vi "CPP_BandLimitBoost.vi"(0 "CutoffFrequencyUsed":dbl=15.0, 3 "CutoffIndex":dbl, 4 "AmplitudeBoost":dbl[](array[numeric])) -> (1 "BandLimitedBoost":dbl[](array[numeric]))   [LabVIEW 2011]
uses:
  <vilib>/Analysis/NI_AALBase.lvlib
panel:
  in  "dF":dbl=0.06103515625
  in  "Combo Box":string(combo)="Cosine"
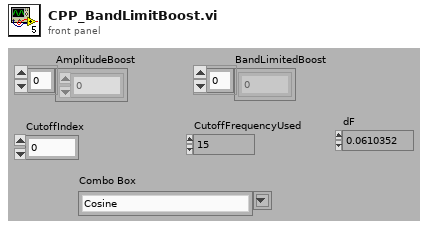
[diagram p1: front panel]
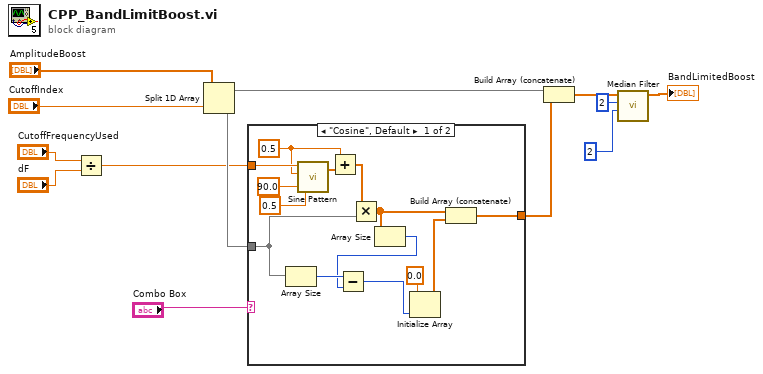
[diagram p0: block diagram]
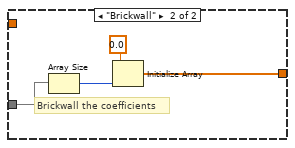
[diagram p2: hidden frame]
diagram:
  n1 = Divide(x="CutoffFrequencyUsed", y="dF") -> (x/y=w5:dbl)
  n2 = Split 1D Array(array="AmplitudeBoost", index="CutoffIndex") -> (first subarray=w11:dbl[], second subarray=w12:dbl[])
  n3 = case shown="\"Cosine\", Default" "Combo Box" {
    tunnel: [w19 w31] -> w13
    tunnel: w12 -> [w21 w29]
    tunnel: w5 -> [w27 _]
    frame "Cosine", Default {
      w22 = 0.5 ("amplitude")
      n4 = Array Size(array=w21) -> (size(s)=w17:i32)
      n5 = call <vilib>:"Sine Pattern.vi"("cycles"=0.5, "phase(degrees)"=90.0, "amplitude"=w22, "samples"=w27) -> ("Sinusoidal Pattern"=w25:dbl[])  [unwired: 1 out]
      n6 = Add(x=w22, y=w25) -> (x+y=w24:dbl[])
      n7 = Multiply(x=w24, y=w21) -> (x*y=w18:dbl[])
      n8 = Array Size(array=w18) -> (size(s)=w16:i32)
      n9 = Subtract(x=w17, y=w16) -> (x-y=w15:i32)
      n10 = Initialize Array(0.0 ("element"), w15) -> (w14:dbl[])
      n11 = Build Array (concatenate)(w18, w14) -> (w19:dbl[])
    }
    frame "Brickwall" {
      # "Brickwall the coefficients"
      n12 = Array Size(array=w29) -> (size(s)=w30:i32)
      n13 = Initialize Array(0.0 ("element"), w30) -> (w31:dbl[])
    }
  }
  n14 = Build Array (concatenate)(w11, w13) -> (w4:dbl[])
  n15 = call <vilib>:"Median Filter.vi"("right rank"=2, "left rank"=2, "X"=w4) -> ("Filtered X"=→"BandLimitedBoost":dbl[])  [unwired: 7 in, 1 out]
